vi "Odour_map_selection_.vi"(10 "Array":i32[](array[numeric]), 11 "Odour component data":T1) -> (3 "input cluster":cluster{"MDS1":dbl[], "MDS2":dbl[]})   [LabVIEW 2016]
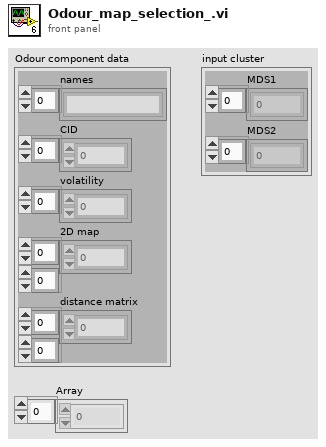
[diagram p1: front panel]
types:
  T1 = cluster{"names":string[], "CID":i32[], "volatility":dbl[], "2D map":dbl[][], "distance matrix":dbl[][]}
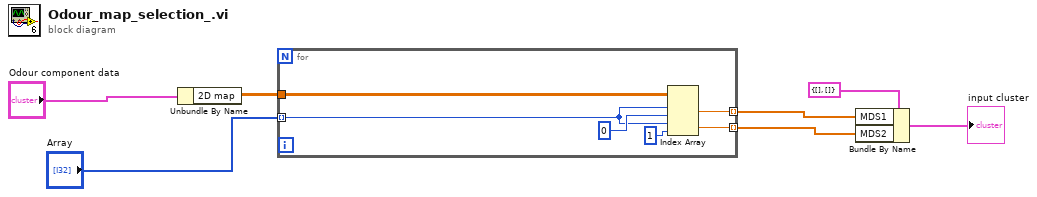
[diagram p0: block diagram]
diagram:
  n1 = Unbundle By Name("Odour component data") -> ("2D map"=w4:dbl[][])
  n2 = for {
    tunnel: w4 -> [w13]
    tunnel: [w12] -> w5 mode=indexing
    tunnel: [w11] -> w6 mode=indexing
    tunnel: "Array" -> [w9] mode=indexing
    n3 = Index Array(array=w13, index (row) #1=w9, index (col) #1=0 ("disabled index (col)"), index (row) #2=w9, index (col) #2=1 ("disabled index (col)")) -> (element #1=w12:dbl, element #2=w11:dbl)
  }
  n4 = Bundle By Name(cluster=cluster{"MDS1":dbl[], "MDS2":dbl[]} {"MDS1"=[], "MDS2"=[]} ("input cluster"), "MDS1"=w5, "MDS2"=w6) -> (→"input cluster":cluster{"MDS1":dbl[], "MDS2":dbl[]})
